vi "Get Terminal Refs for New Frame.vi"(8 "error in (no error)":errorcluster, 10 "Case Structure Ref":refnum<vi>, 11 "Setter Generator In":refnum<class "API VI Generator.lvclass">) -> (0 "error out":errorcluster, 2 "reference out":refnum<vi>, 3 "Setter Generator Out":refnum<class "API VI Generator.lvclass">)   [LabVIEW 2020, in "Method Generation.lvlib" / "API VI Generator.lvclass"]
uses:
  API VI Generator.lvclass
  API VI Generator.lvclass/API VI Generator.ctl
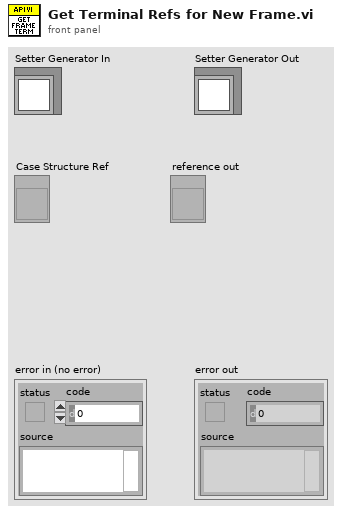
[diagram p1: front panel]
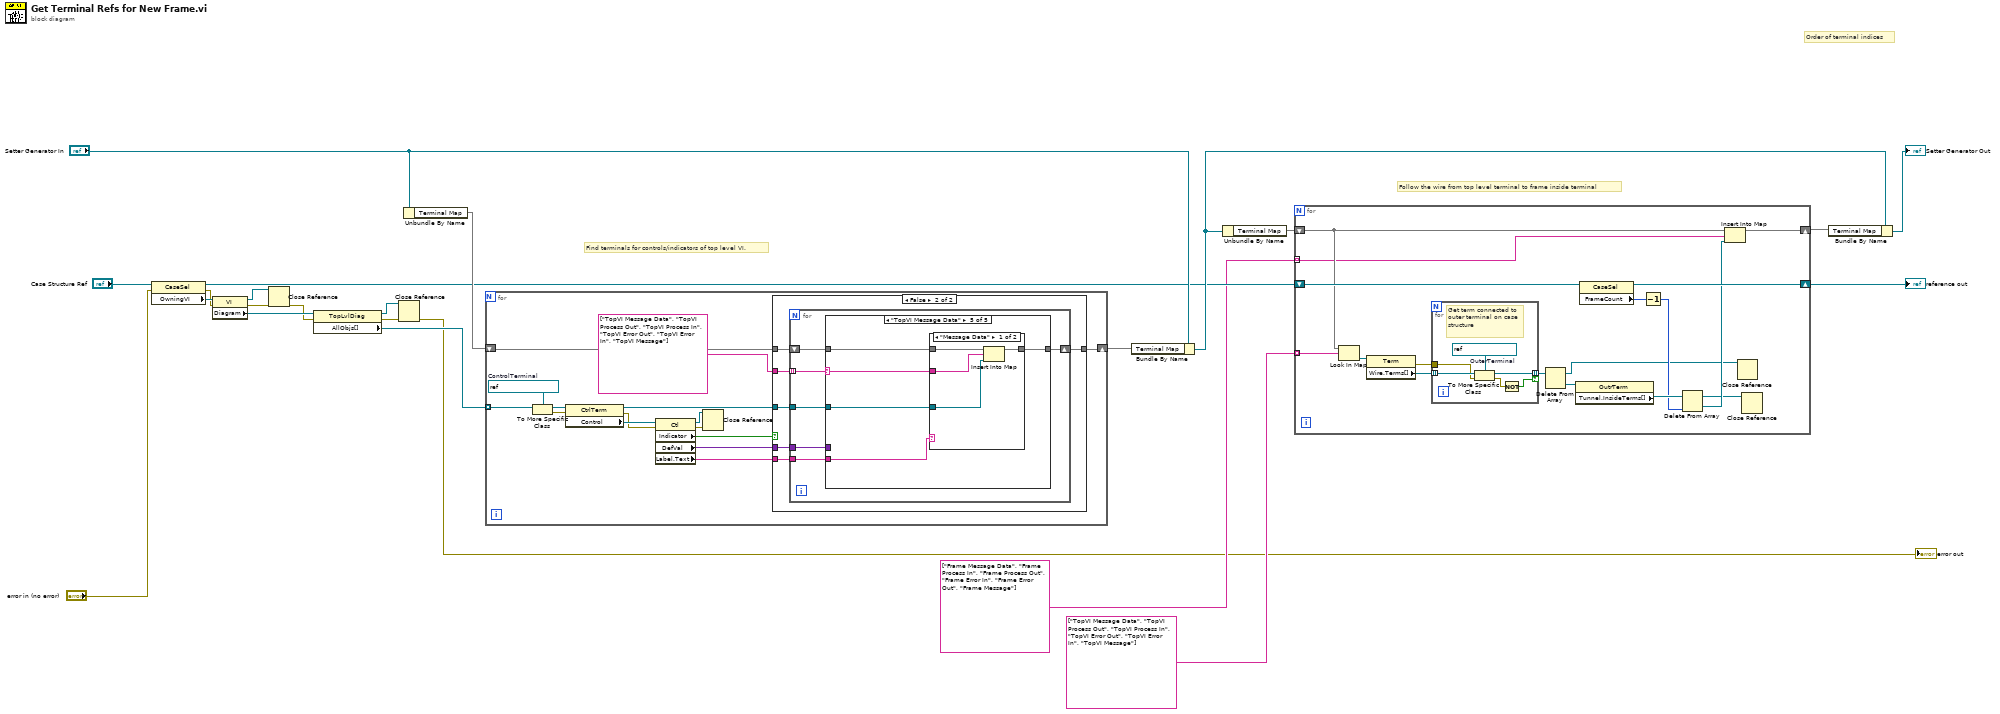
[diagram p0: block diagram]
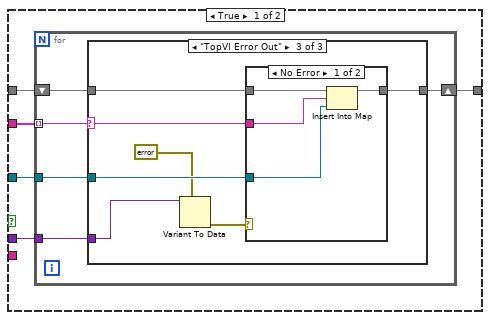
[diagram p2: hidden frame]
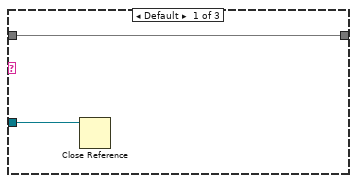
[diagram p3: hidden frame]
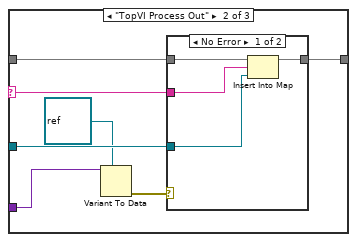
[diagram p4: hidden frame]
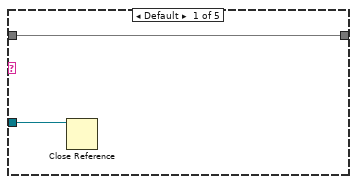
[diagram p7: hidden frame]
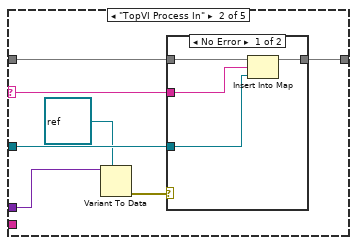
[diagram p8: hidden frame]
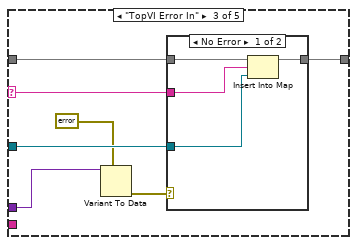
[diagram p10: hidden frame]
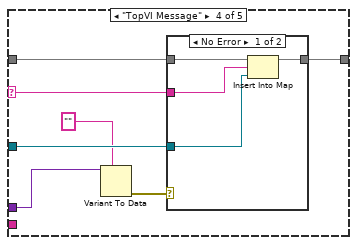
[diagram p12: hidden frame]
diagram:
  # "Follow the wire from top level terminal to frame inside terminal"
  # "Find terminals for controls/indicators of top level VI."
  # "Order of terminal indices"
  n1 = property class="CaseSel"(reference="Case Structure Ref", error in="error in (no error)") -> (reference out=w13:refnum<vi>, error out=w17:errorcluster, "OwningVI"=w23:refnum<vi>)
  n2 = property class="VI"(reference=w23, error in=w17) -> (reference out=w4:refnum<vi>, error out=w16:errorcluster, "Diagram"=w21:refnum<vi>)
  n3 = Close Reference(reference=w4, error in (no error)=w16) -> (error out=w5:errorcluster)
  n4 = property class="TopLvlDiag"(reference=w21, error in=w5) -> (reference out=w2:refnum<vi>, error out=w3:errorcluster, "AllObjs[]"=w22:refnum<vi>[])
  n5 = Close Reference(reference=w2, error in (no error)=w3) -> (error out=→"error out":errorcluster)
  n6 = Unbundle By Name("Setter Generator In") -> ("Terminal Map"=w18:map{string, refnum<vi>})
  n7 = for {
    tunnel: w22 -> [w36] mode=indexing
    shift-right: [w37] -> w7
    shift-left: w18 -> [w38]
    w34 = refnum<vi> refnum  # ControlTerminal
    n8 = To More Specific Class(target class=w34, reference=w36) -> (specific class reference=w35:refnum<vi>, error out=w28:errorcluster)  [unwired: 1 in]
    n9 = property class="CtrlTerm"(reference=w35, error in=w28) -> (reference out=w33:refnum<vi>, error out=w27:errorcluster, "Control"=w32:refnum<vi>)
    n10 = property class="Ctl"(reference=w32, error in=w27) -> (reference out=w25:refnum<vi>, error out=w26:errorcluster, "Indicator"=w31:bool, "DefVal"=w30:variant, "Label.Text"=w24:string)
    n11 = Close Reference(reference=w25, error in (no error)=w26) -> ()  [unwired: 1 out]
    n12 = case shown="False" w31 {
      tunnel: w38 -> [w43 w80]
      tunnel: [w42 w79] -> w37
      tunnel: w33 -> [w41 w78]
      tunnel: w30 -> [w40 w77]
      tunnel: string[] ["TopVI Message Data", "TopVI Process Out", "TopVI Process In", "TopVI Error Out", "TopVI Error In", "TopVI Message"] ("Array") -> [w39 w76]
      tunnel: w24 -> [_ w75]
      frame True {
        n13 = for {
          tunnel: w41 -> [w46]
          tunnel: w40 -> [w45]
          shift-right: [w47] -> w42
          shift-left: w43 -> [w48]
          tunnel: w39 -> [w44] mode=indexing
          n14 = case shown="\"TopVI Error Out\"" w44 {
            selector: w44 -> [_ w53 w65]
            tunnel: w48 -> [w50 w57 w69]
            tunnel: [w50 w56 w68] -> w47
            tunnel: w46 -> [w49 w55 w67]
            tunnel: w45 -> [_ w54 w66]
            frame Default {
              n15 = Close Reference(reference=w49) -> ()  [unwired: 1 in, 1 out]
            }
            frame "TopVI Process Out" {
              n16 = Variant To Data(type=refnum<class> refnum ("LabVIEW Object"), Variant=w54) -> (error out=w51:errorcluster)  [unwired: 1 in, 1 out]
              n17 = case shown="No Error" w51 {
                tunnel: w57 -> [w61 w62]
                tunnel: [w60 w62] -> w56
                tunnel: w55 -> [w59 _]
                tunnel: w53 -> [w58 _]
                frame No Error {
                  n18 = Insert Into Map(map in=w61, key=w58, value=w59) -> (map out=w60:map{string, refnum<vi>})  [unwired: 2 out]
                }
                frame Error {
                }
              }
            }
            frame "TopVI Error Out" {
              n19 = Variant To Data(type=errorcluster {"status"=FALSE, "code"=0, "source"=""} ("error constant"), Variant=w66) -> (error out=w63:errorcluster)  [unwired: 1 in, 1 out]
              n20 = case shown="No Error" w63 {
                tunnel: w69 -> [w73 w74]
                tunnel: [w72 w74] -> w68
                tunnel: w67 -> [w71 _]
                tunnel: w65 -> [w70 _]
                frame No Error {
                  n21 = Insert Into Map(map in=w73, key=w70, value=w71) -> (map out=w72:map{string, refnum<vi>})  [unwired: 2 out]
                }
                frame Error {
                }
              }
            }
          }
        }
      }
      frame False {
        n22 = for {
          tunnel: w78 -> [w84]
          tunnel: w77 -> [w83]
          shift-right: [w85] -> w79
          shift-left: w80 -> [w86]
          tunnel: w76 -> [w82] mode=indexing
          tunnel: w75 -> [w81]
          n23 = case shown="\"TopVI Message Data\"" w82 {
            selector: w82 -> [_ w91 w103 w115 w126]
            tunnel: w86 -> [w88 w95 w107 w119 w129]
            tunnel: [w88 w94 w106 w118 w128] -> w85
            tunnel: w84 -> [w87 w93 w105 w117 w127]
            tunnel: w83 -> [_ w92 w104 w116 _]
            tunnel: w81 -> [_ _ _ _ w125]
            frame Default {
              n24 = Close Reference(reference=w87) -> ()  [unwired: 1 in, 1 out]
            }
            frame "TopVI Process In" {
              n25 = Variant To Data(type=refnum<class> refnum ("LabVIEW Object"), Variant=w92) -> (error out=w89:errorcluster)  [unwired: 1 in, 1 out]
              n26 = case shown="No Error" w89 {
                tunnel: w95 -> [w99 w100]
                tunnel: [w98 w100] -> w94
                tunnel: w93 -> [w97 _]
                tunnel: w91 -> [w96 _]
                frame No Error {
                  n27 = Insert Into Map(map in=w99, key=w96, value=w97) -> (map out=w98:map{string, refnum<vi>})  [unwired: 2 out]
                }
                frame Error {
                }
              }
            }
            frame "TopVI Error In" {
              n28 = Variant To Data(type=errorcluster {"status"=FALSE, "code"=0, "source"=""} ("error constant"), Variant=w104) -> (error out=w101:errorcluster)  [unwired: 1 in, 1 out]
              n29 = case shown="No Error" w101 {
                tunnel: w107 -> [w111 w112]
                tunnel: [w110 w112] -> w106
                tunnel: w105 -> [w109 _]
                tunnel: w103 -> [w108 _]
                frame No Error {
                  n30 = Insert Into Map(map in=w111, key=w108, value=w109) -> (map out=w110:map{string, refnum<vi>})  [unwired: 2 out]
                }
                frame Error {
                }
              }
            }
            frame "TopVI Message" {
              n31 = Variant To Data(type="" ("error constant"), Variant=w116) -> (error out=w113:errorcluster)  [unwired: 1 in, 1 out]
              n32 = case shown="No Error" w113 {
                tunnel: w119 -> [w123 w124]
                tunnel: [w122 w124] -> w118
                tunnel: w117 -> [w121 _]
                tunnel: w115 -> [w120 _]
                frame No Error {
                  n33 = Insert Into Map(map in=w123, key=w120, value=w121) -> (map out=w122:map{string, refnum<vi>})  [unwired: 2 out]
                }
                frame Error {
                }
              }
            }
            frame "TopVI Message Data" {
              n34 = case shown="\"Message Data\"" w125 {
                tunnel: w129 -> [w133 w134]
                tunnel: [w132 w134] -> w128
                tunnel: w127 -> [w131 _]
                tunnel: w126 -> [w130 _]
                frame "Message Data" {
                  n35 = Insert Into Map(map in=w133, key=w130, value=w131) -> (map out=w132:map{string, refnum<vi>})  [unwired: 2 out]
                }
                frame Default {
                }
              }
            }
          }
        }
      }
    }
  }
  n36 = Bundle By Name(cluster="Setter Generator In", "Terminal Map"=w7) -> (w14:refnum<class "API VI Generator.lvclass">)
  n37 = Unbundle By Name(w14) -> ("Terminal Map"=w11:map{string, refnum<vi>})
  n38 = for {
    shift-right: [w142] -> w12
    shift-left: w13 -> [w145]
    shift-right: [w138] -> w8
    shift-left: w11 -> [w141]
    tunnel: string[] ["TopVI Message Data", "TopVI Process Out", "TopVI Process In", "TopVI Error Out", "TopVI Error In", "TopVI Message"] ("Array") -> [w140] mode=indexing
    tunnel: string[] ["Frame Message Data", "Frame Process In", "Frame Process Out", "Frame Error In", "Frame Error Out", "Frame Message"] -> [w139] mode=indexing
    n39 = Look In Map(map=w141, key=w140) -> (value=w151:refnum<vi>)  [unwired: 1 in, 1 out]
    n40 = property class="Term"(reference=w151) -> (error out=w149:errorcluster, "Wire.Terms[]"=w150:refnum<vi>[])  [unwired: 1 in, 1 out]
    n41 = for {
      tunnel: w150 -> [w157] mode=indexing
      tunnel: [w155] -> w148 mode=indexing if=w153
      tunnel: w149 -> [w152]
      w156 = refnum<vi> refnum  # OuterTerminal
      # "Get term connected to outer terminal on case structure"
      n42 = To More Specific Class(target class=w156, reference=w157, error in=w152) -> (specific class reference=w155:refnum<vi>, error out=w154:errorcluster)
      n43 = Not(x=w154) -> (.not. x?=w153:bool)
    }
    n44 = Delete From Array(array=w148) -> (deleted portion=w147:refnum<vi>, array with subset deleted=w135:refnum<vi>[])  [unwired: 2 in]
    n45 = property class="OutrTerm"(reference=w147) -> ("Tunnel.InsideTerms[]"=w146:refnum<vi>[])  [unwired: 1 in, 2 out]
    n46 = property class="CaseSel"(reference=w145) -> (reference out=w142:refnum<vi>, "FrameCount"=w144:i32)  [unwired: 1 in, 1 out]
    n47 = Decrement(x=w144) -> (x-1=w143:i32)
    n48 = Delete From Array(array=w146, index=w143) -> (deleted portion=w137:refnum<vi>, array with subset deleted=w136:refnum<vi>[])  [unwired: 1 in]
    n49 = Insert Into Map(map in=w141, key=w139, value=w137) -> (map out=w138:map{string, refnum<vi>})  [unwired: 2 out]
    n50 = Close Reference(reference=w135) -> ()  [unwired: 1 in, 1 out]
    n51 = Close Reference(reference=w136) -> ()  [unwired: 1 in, 1 out]
  }
  "reference out" <- w12
  n52 = Bundle By Name(cluster=w14, "Terminal Map"=w8) -> (→"Setter Generator Out":refnum<class "API VI Generator.lvclass">)
